vi "Finalize Settings 1.0.vi"(8 "error in (no error)":errorcluster, 11 "configuration 1.0":T1={"name"="Group", "direction"=enum."Tx", "cycle timing"={"priority"=100, "decimation"=1, "offset"=0}, "timeout behavior"=enum."Increment Late Count"}) -> (0 "error out":errorcluster, 2 "settings version":T2, 3 "settings":cluster{"key":string, "value":string}[](array[cluster]))   [LabVIEW 2017, in "DSF Core.lvlib" / "Core Group Configuration.lvclass"]
uses:
  Core Group Configuration.lvclass
  Typedefs/DSF Version Info.ctl
  DSF Core.lvlib
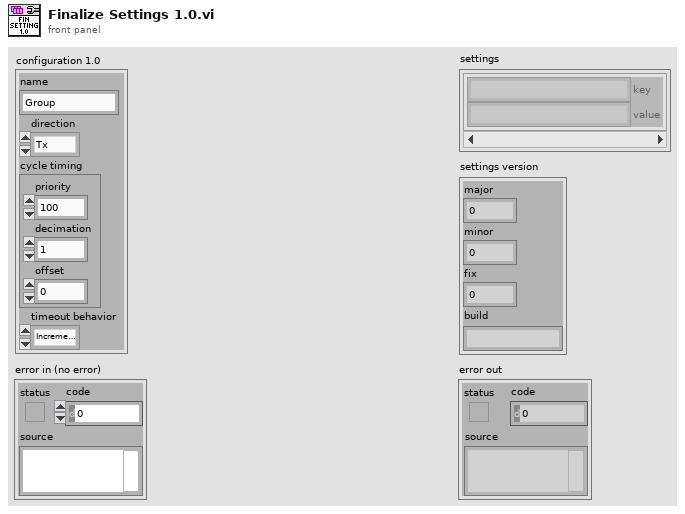
[diagram p1: front panel]
types:
  T1 = cluster{"name":string, "direction":enum8{"Tx", "Rx"}, "cycle timing":cluster{"priority":u64, "decimation":u64, "offset":u64}, "timeout behavior":enum8{"Increment Late Count", "Throw Error"}}
  T2 = typedef "DSF Core.lvlib/DSF Version Info.ctl" = cluster{"major":u32, "minor":u32, "fix":u32, "build":string}
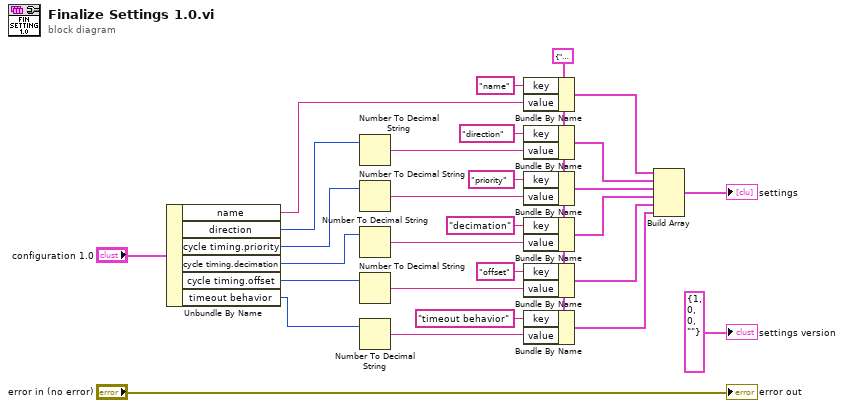
[diagram p0: block diagram]
diagram:
  w4 = cluster{"key":string, "value":string} {"key"="", "value"=""} ("setting")
  n1 = Unbundle By Name("configuration 1.0") -> ("name"=w19:string, "direction"=w10:enum8{"Tx", "Rx"}, "cycle timing.priority"=w15:u64, "cycle timing.decimation"=w14:u64, "cycle timing.offset"=w13:u64, "timeout behavior"=w6:enum8{"Increment Late Count", "Throw Error"})
  n2 = Number To Decimal String(number=w10) -> (decimal integer string=w9:string)  [unwired: 1 in]
  n3 = Number To Decimal String(number=w15) -> (decimal integer string=w18:string)  [unwired: 1 in]
  n4 = Number To Decimal String(number=w14) -> (decimal integer string=w17:string)  [unwired: 1 in]
  n5 = Number To Decimal String(number=w13) -> (decimal integer string=w16:string)  [unwired: 1 in]
  n6 = Number To Decimal String(number=w6) -> (decimal integer string=w3:string)  [unwired: 1 in]
  n7 = Bundle By Name(cluster=w4, "key"="name", "value"=w19) -> (w28:cluster{"key":string, "value":string})
  n8 = Bundle By Name(cluster=w4, "key"="direction", "value"=w9) -> (w27:cluster{"key":string, "value":string})
  n9 = Bundle By Name(cluster=w4, "key"="priority", "value"=w18) -> (w26:cluster{"key":string, "value":string})
  n10 = Bundle By Name(cluster=w4, "key"="decimation", "value"=w17) -> (w25:cluster{"key":string, "value":string})
  n11 = Bundle By Name(cluster=w4, "key"="offset", "value"=w16) -> (w12:cluster{"key":string, "value":string})
  n12 = Bundle By Name(cluster=w4, "key"="timeout behavior", "value"=w3) -> (w2:cluster{"key":string, "value":string})
  n13 = Build Array(w28, w27, w26, w25, w12, w2) -> (→"settings":cluster{"key":string, "value":string}[])
  "error out" <- "error in (no error)"
  "settings version" <- T2 {"major"=1, "minor"=0, "fix"=0, "build"=""} ("settings version")
